vi "ThresholdLevelFinder.vi"(6 "Initial Threshold":i32=100, 7 "Channel":u32=2, 8 "error in (no error)":errorcluster, 9 "id_in":i32, 10 "connection ID":refnum<k5>, 11 "VISA resource name":refnum<visa-resource-name>="Oscilloscope") -> (0 "error out":errorcluster, 1 "id_out":i32, 2 "connection ID out":refnum<k5>, 3 "VISA resource name out":refnum<visa-resource-name>="Oscilloscope", 4 "threshold out":i32=470)   [LabVIEW 2009]
panel:
  in  "increment":i32=10
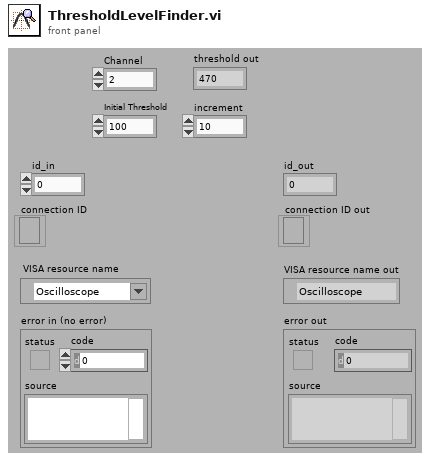
[diagram p1: front panel]
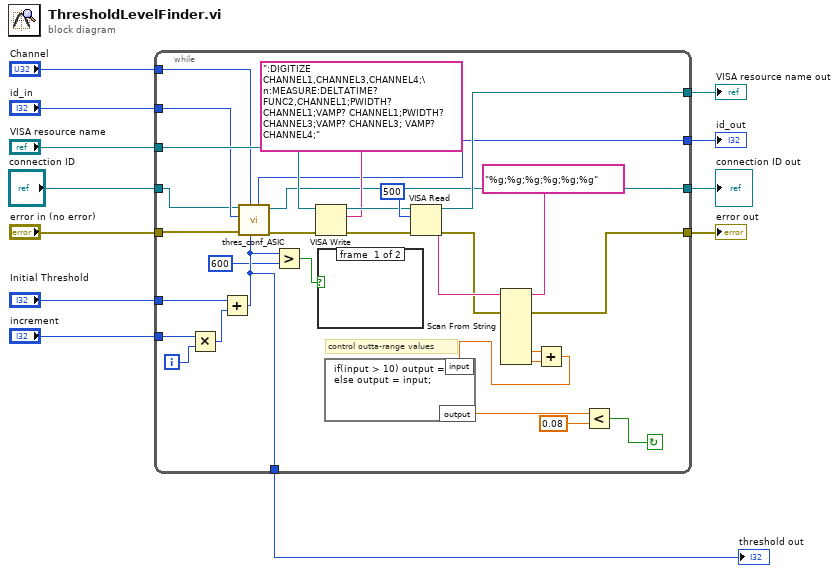
[diagram p0: block diagram]
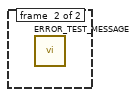
[diagram p2: hidden frame]
diagram:
  n1 = while {
    tunnel: "VISA resource name" -> [w32]
    tunnel: [w31] -> w11
    tunnel: "connection ID" -> [w14]
    tunnel: [w30] -> w9
    tunnel: [w29] -> w8
    tunnel: "error in (no error)" -> [w13]
    tunnel: "id_in" -> [w24]
    tunnel: [w23] -> w5
    tunnel: "Channel" -> [w22]
    tunnel: [w17] -> w3
    tunnel: "Initial Threshold" -> [w21]
    tunnel: "increment" -> [w20]
    i -> [w26]
    stop <- w28 continue-if-true
    # "control outta-range values"
    n2 = Multiply(x=w20, y=w26) -> (x*y=w25:i32)
    n3 = Add(x=w21, y=w25) -> (x+y=w17:i32)
    n4 = call "thres_conf_ASIC.vi"("threshold"=w17, "Ring"=w22, "error out 3"=w13, "Id in"=w24, "connection ID"=w14) -> ("error out 2"=w33:errorcluster, "connection ID out"=w30:refnum<k5>, "Id out"=w23:i32)  [unwired: 3 in, 1 out]
    n5 = Greater?(x=w17, y=600) -> (0:w15:bool)
    n6 = VISA Write(VISA resource name=w32, write buffer=":DIGITIZE CHANNEL1,CHANNEL3,CHANNEL4;\n:MEASURE:DELTATIME? FUNC2,CHANNEL1;PWIDTH? CHANNEL1;VAMP? CHANNEL1;PWIDTH? CHANNEL3;VAMP? CHANNEL3; VAMP? CHANNEL4;", error in (no error)=w33) -> (VISA resource name out=w37:refnum<visa-resource-name>, error out=w38:errorcluster)  [unwired: 1 out]
    n7 = case shown="True" w15 {
      frame #0 {
      }
      frame #1 {
        n8 = call "ERROR_TEST_MESSAGE.vi"() -> ()  [unwired: 11 in, 1 out]
      }
    }
    n9 = VISA Read(VISA resource name=w37, byte count=u32 500, error in (no error)=w38) -> (VISA resource name out=w31:refnum<visa-resource-name>, read buffer=w41:string, error out=w39:errorcluster)  [unwired: 1 out]
    n10 = Scan From String(format string="%g;%g;%g;%g;%g;%g", input string=w41, error in=w39) -> (error out=w29:errorcluster, output 5=w35:dbl, output 6=w34:dbl)  [unwired: 11 in, 2 out]
    n11 = Add(x=w35, y=w34) -> (x+y=w18:dbl)
    n12 = formula code="if(input > 10) output = 0.0;\nelse output = input;"("input"=w18) -> ("output"=w19:dbl)
    n13 = Less?(x=w19, y=0.08) -> (x < y?=w28:bool)
  }
  "VISA resource name out" <- w11
  "error out" <- w8
  "connection ID out" <- w9
  "id_out" <- w5
  "threshold out" <- w3
